vi "PRAMMS-LISTENER.vi"(0 "PRAMMS-COMM IN":refnum<visa-resource-name>="Yp\u0000\u0002", 1 "Bool Refnum":refnum<vi>, 2 "MessageTypeArray":cluster{string[], u32[]}={["emtError", "emtAreYouThere", "emtAcknowledgment", "emtGetClientType", "emtClientType", "emtGetImageExposureTime", "emtSetImageExposureTime", "emtImageExposureTime", "emtGetOptimalExposureTime", "emtSetOptimalExposureTime", "emtOptimalExposureTime", "emtGetImageEMGain", "emtSetImageEMGain", "emtImageEMGain", "emtGetFPGACtrl", "emtSetFPGACtrl", "emtFPGACtrl", "emtGetImageWidth", "emtSetImageWidth", "emtImageWidth", "emtGetImageHeight", "emtSetImageHeight", "emtImageHeight", "emtGetImageBinning", "emtSetImageBinning", "emtImageBinning", "emtGetImageDisplayFrameRate", "emtSetImageDisplayFrameRate", "emtImageDisplayFrameRate", "emtGetROIWidth", "emtSetROIWidth", "emtROIWidth", "emtGetROIHeight", "emtSetROIHeight", "emtROIHeight", "emtGetROIXOffset", "emtSetROIXOffset", "emtROIXOffset", "emtGetROIYOffset", "emtSetROIYOffset", "emtROIYOffset", "emtStartAcquisition", "mtStopAcquisition", "emtAcquisitionStarted", "emtAcquisitionStopped", "emtGetFalconImage", "emtFalconImage"], [1, 2, 3, 4, 5, 1001, 1101, 1201, 1002, 1102, 1202, 1003, 1103, 1203, 1004, 1104, 1204, 1005, 1105, 1205, 1006, 1106, 1206, 1007, 1107, 1207, 1008, 1108, 1208, 1009, 1109, 1209, 1010, 1110, 1210, 1011, 1111, 1211, 1012, 1112, 1212, 1130, 1131, 1150, 1151, 1070, 1270]}, 7 "Signature":u32=1886544237, 11 "Error IN":errorcluster, 12 "ReadTimeOut":i32=5) -> (4 "PRAMMS-COMM OUT":refnum<visa-resource-name>, 6 "Type":string, 8 "Received":timestamp, 10 "ByteArray":u8[](array[numeric]), 14 "Received?":bool, 15 "Error OUT":errorcluster)   [LabVIEW 2019]
panel:
  out "DataReadTime":u32
  out "HeaderTime":u32
  out "Wait4FlagTime":u32=16
  out "MessageLength":u32
  out "CommandEnum":string[](array[string])=["emtError", "emtAreYouThere", "emtAcknowledgment", "emtGetClientType", "emtClientType", "emtGetImageExposureTime", "emtSetImageExposureTime", "emtImageExposureTime", "emtGetOptimalExposureTime", "emtSetOptimalExposureTime", "emtOptimalExposureTime", "emtGetImageEMGain", "emtSetImageEMGain", "emtImageEMGain", "emtGetFPGACtrl", "emtSetFPGACtrl", "emtFPGACtrl", "emtGetImageWidth", "emtSetImageWidth", "emtImageWidth", "emtGetImageHeight", "emtSetImageHeight", "emtImageHeight", "emtGetImageBinning", "emtSetImageBinning", "emtImageBinning", "emtGetImageDisplayFrameRate", "emtSetImageDisplayFrameRate", "emtImageDisplayFrameRate", "emtGetROIWidth", "emtSetROIWidth", "emtROIWidth", "emtGetROIHeight", "emtSetROIHeight", "emtROIHeight", "emtGetROIXOffset", "emtSetROIXOffset", "emtROIXOffset", "emtGetROIYOffset", "emtSetROIYOffset", "emtROIYOffset", "emtStartAcquisition", "mtStopAcquisition", "emtAcquisitionStarted", "emtAcquisitionStopped", "emtGetFalconImage", "emtFalconImage"]
  out "TypeEnum":u32[](array[numeric])=[1, 2, 3, 4, 5, 1001, 1101, 1201, 1002, 1102, 1202, 1003, 1103, 1203, 1004, 1104, 1204, 1005, 1105, 1205, 1006, 1106, 1206, 1007, 1107, 1207, 1008, 1108, 1208, 1009, 1109, 1209, 1010, 1110, 1210, 1011, 1111, 1211, 1012, 1112, 1212, 1130, 1131, 1150, 1151, 1070, 1270]
  # "Ce programme sera mis dans une boucle de communication \"ininterrompable\"\n\nIl doit toujours écouter la connexion si elle existe et retourne le EnumMessageTYpe\net le data string s'il existe.  Ainsi, quand il recevra un ACK, il retournera le code du\n\"emtAcknoledgment\" vers le programme principal qui s'occuppera de lever le flag.\n\nSon éxécution devra être suivi d'une boucle d'interprétation qui appelera le bon vi\nd'interprétation en fonction du MessageType reçu."
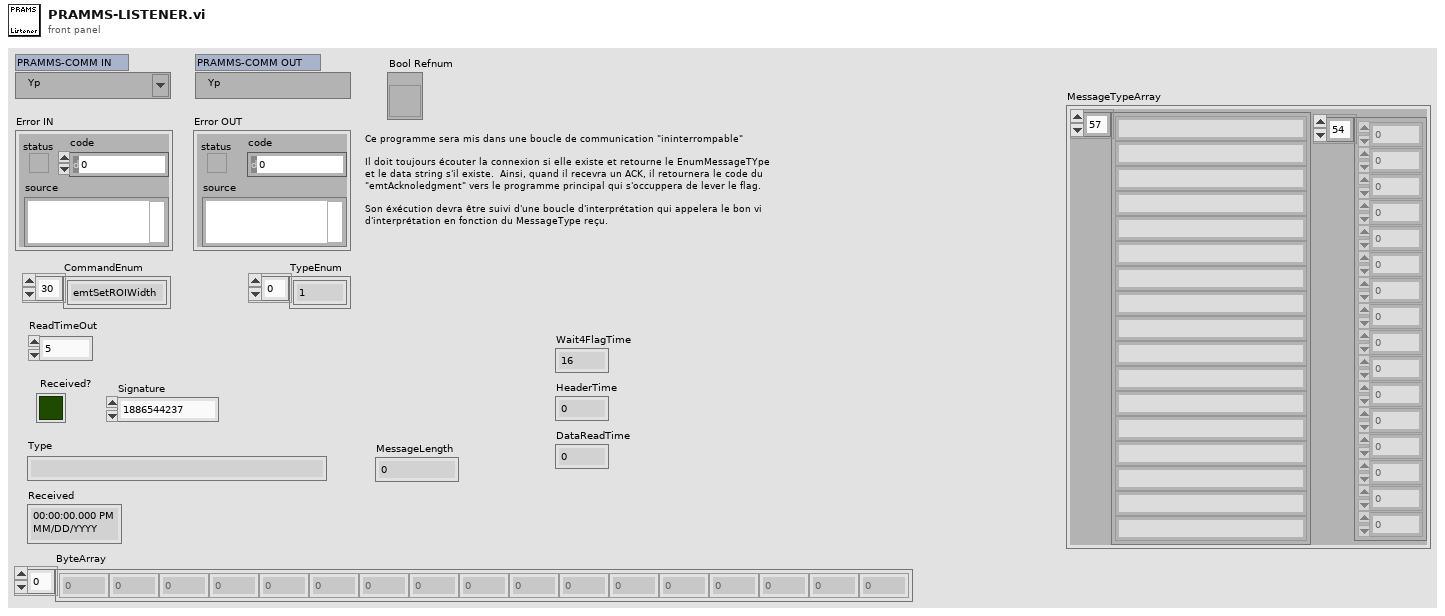
[diagram p1: front panel]
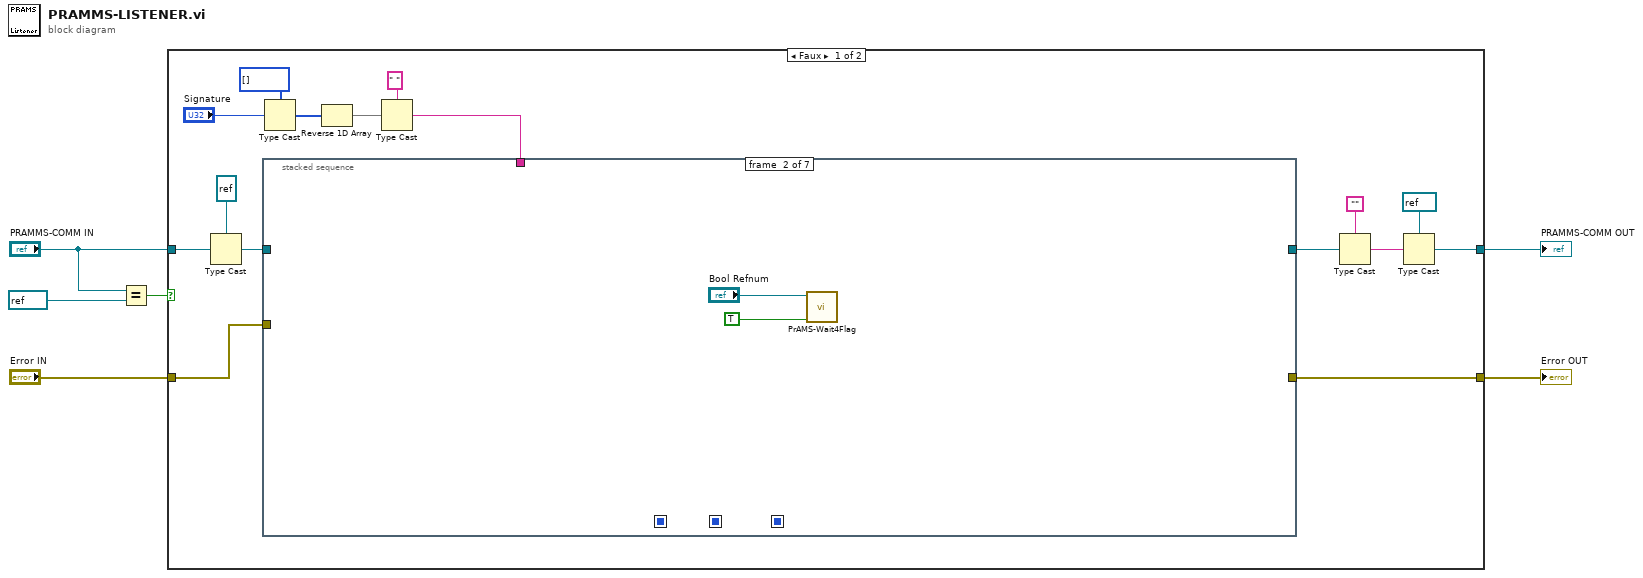
[diagram p0: block diagram]
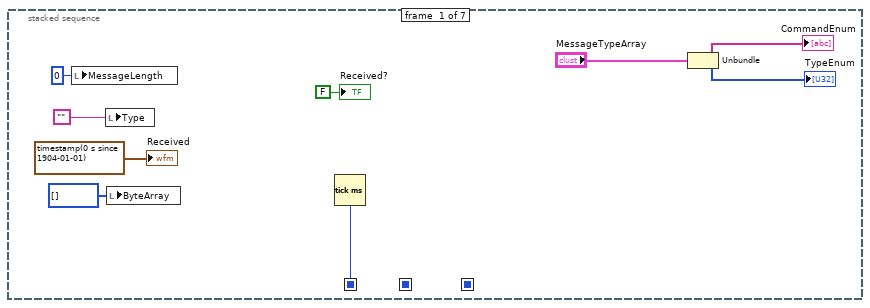
[diagram p2: hidden frame]
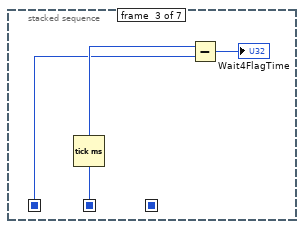
[diagram p3: hidden frame]
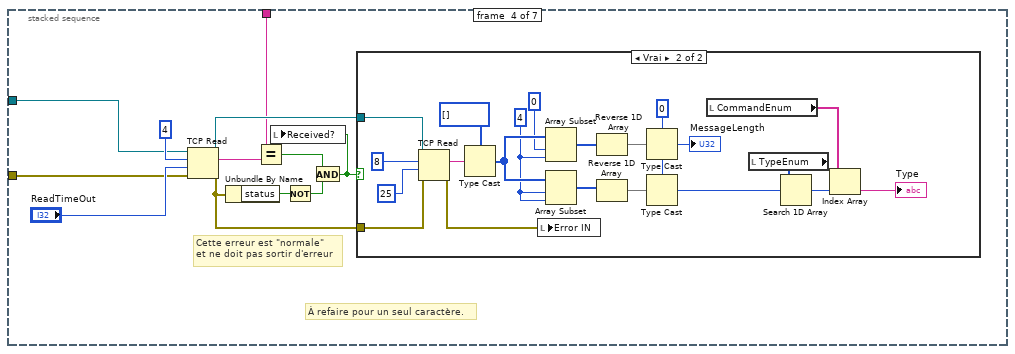
[diagram p4: hidden frame]
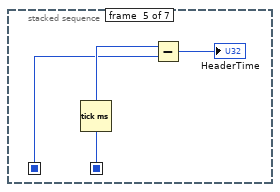
[diagram p6: hidden frame]
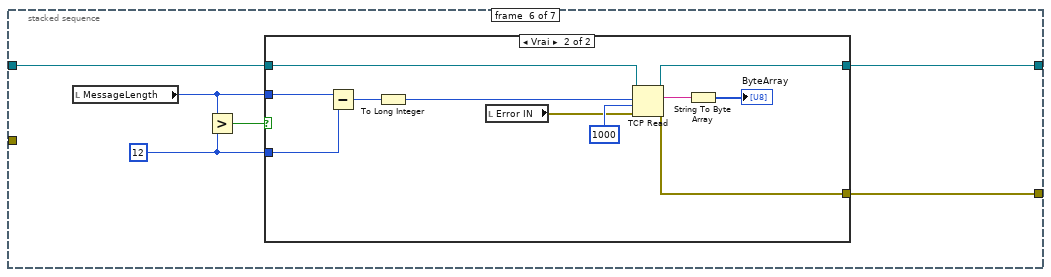
[diagram p7: hidden frame]
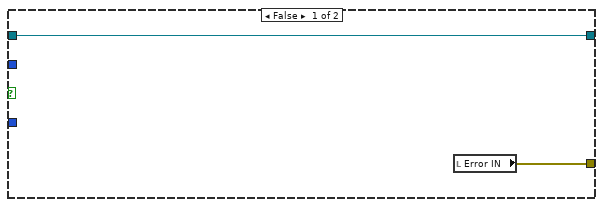
[diagram p8: hidden frame]
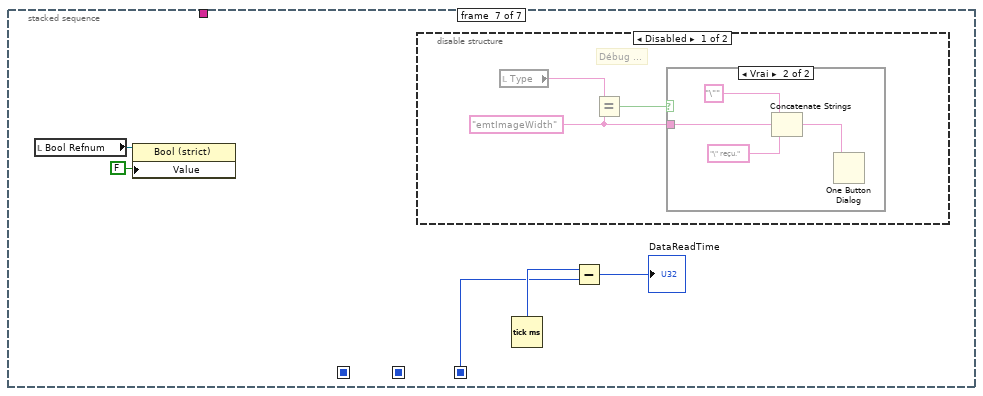
[diagram p9: hidden frame]
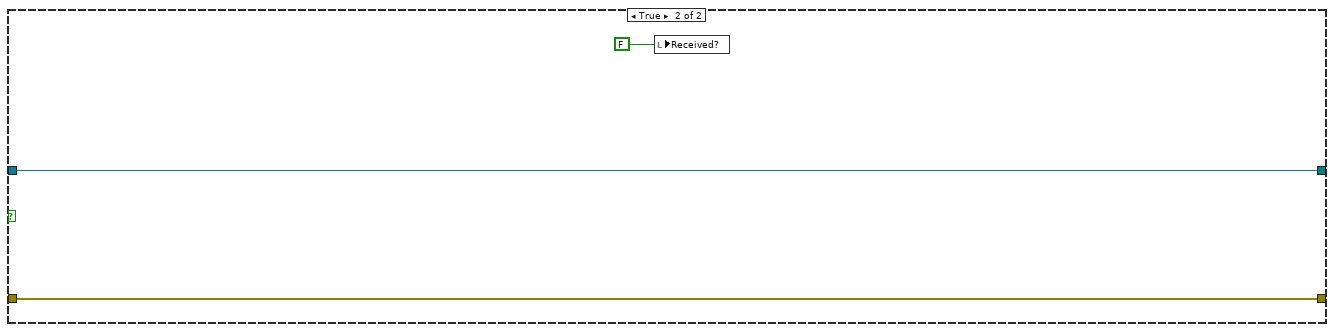
[diagram p12: hidden frame]
diagram:
  n1 = Equal?(x="PRAMMS-COMM IN", y=refnum<visa-resource-name> "-1") -> (x = y?=w5:bool)
  n2 = case shown="Faux" w5 {
    tunnel: "PRAMMS-COMM IN" -> [w22 w106]
    tunnel: "Error IN" -> [w19 w105]
    tunnel: [w14 w106] -> w1
    tunnel: [w18 w105] -> w2
    frame False {
      n3 = Type Cast(type=refnum<k5> refnum ("connection ID"), x=w22) -> (*(type *) &x=w21:refnum<k5>)
      n4 = Type Cast(type=u8[] [], x="Signature") -> (*(type *) &x=w12:u8[])
      n5 = Reverse 1D Array(array=w12) -> (reversed array=w9:u8[])
      n6 = Type Cast(type=" ", x=w9) -> (*(type *) &x=w7:string)
      n7 = stacked-sequence {
        seq-local: [w27 _ _ _ _ _ _] -> [_ _ w34 _ _ _ _]
        seq-local: [_ _ w35 _ _ _ _] -> [_ _ _ _ w70 _ _]
        seq-local: [_ _ _ _ w71 _ _] -> [_ _ _ _ _ _ w92]
        tunnel: w21 -> [_ _ _ w40 _ w75 _]
        tunnel: w19 -> [_ _ _ w39 _ _ _]
        tunnel: [_ _ _ _ _ w74 _] -> w18
        tunnel: [_ _ _ _ _ w73 _] -> w13
        tunnel: w7 -> [_ _ _ w38 _ _ _]
        frame #0 {
          n8 = local write "MessageLength"(u32 0 ("MessageLength")) -> ()
          n9 = local write "Type"("") -> ()
          n10 = local write "ByteArray"(u8[] [] ("ByteArray")) -> ()
          n11 = Tick Count (ms)() -> (millisecond timer value=w27:u32)
          n12 = Unbundle("MessageTypeArray") -> (→"CommandEnum":string[], →"TypeEnum":u32[])
          "Received?" <- FALSE ("RCV")
          "Received" <- timestamp(0 s since 1904-01-01) ("Received")
        }
        frame #1 {
          n13 = call "PrAMS-Wait4Flag.vi"("Raise Flag ?"=TRUE, "Ctl Refnum IN"="Bool Refnum") -> ()  [unwired: 8 in, 2 out]
        }
        frame #2 {
          n14 = Tick Count (ms)() -> (millisecond timer value=w35:u32)
          n15 = Subtract(x=w35, y=w34) -> (x-y=→"Wait4FlagTime":u32)
        }
        frame #3 {
          # "À refaire pour un seul caractère."
          # "Cette erreur est \"normale\"\net ne doit pas sortir d'erreur"
          n16 = TCP Read(connection ID=w40, bytes to read=4, error in (no error)=w39, 9:"ReadTimeOut") -> (connection ID out=w42:refnum<k5>, data out=w46:string, error out=w43:errorcluster)  [unwired: 1 in]
          n17 = Unbundle By Name(w43) -> ("status"=w44:bool)
          n18 = Equal?(x=w38, y=w46) -> (x = y?=w45:bool)
          n19 = Not(x=w44) -> (.not. x?=w37:bool)
          n20 = And(x=w45, y=w37) -> (x .and. y?=w41:bool)
          n21 = local write "Received?"(w41) -> ()
          n22 = case shown="Vrai" w41 {
            tunnel: w43 -> [_ w68]
            tunnel: w42 -> [_ w69]
            frame False {
            }
            frame True {
              w56 = u32 0
              w60 = 4 ("length")
              n23 = TCP Read(connection ID=w69, bytes to read=8, error in (no error)=w68, 9:25 ("timeout ms (25000)")) -> (data out=w63:string, error out=w49:errorcluster)  [unwired: 1 in, 1 out]
              n24 = Type Cast(type=u8[] [], x=w63) -> (*(type *) &x=w61:u8[])
              n25 = local write "Error IN"(w49) -> ()
              n26 = Array Subset(array=w61, index=0, length=w60) -> (w64:u8[])
              n27 = Array Subset(array=w61, index=w60, length=w60) -> (w65:u8[])
              n28 = Reverse 1D Array(array=w64) -> (reversed array=w59:u8[])
              n29 = Reverse 1D Array(array=w65) -> (reversed array=w57:u8[])
              n30 = Type Cast(type=w56, x=w59) -> (*(type *) &x=→"MessageLength":u32)
              n31 = Type Cast(type=w56, x=w57) -> (*(type *) &x=w54:u32)
              n32 = local read "CommandEnum"() -> (w52:string[])
              n33 = local read "TypeEnum"() -> (w53:u32[])
              n34 = Search 1D Array(1D array=w53, element=w54) -> (index of element=w50:i32)  [unwired: 1 in]
              n35 = Index Array(array=w52, index=w50) -> (element=→"Type":string)
            }
          }
        }
        frame #4 {
          n36 = Tick Count (ms)() -> (millisecond timer value=w71:u32)
          n37 = Subtract(x=w71, y=w70) -> (x-y=→"HeaderTime":u32)
        }
        frame #5 {
          w76 = u32 12 ("y")
          n38 = local read "MessageLength"() -> (w77:u32)
          n39 = Greater?(x=w77, y=w76) -> (0:w78:bool)
          n40 = case shown="Vrai" w78 {
            tunnel: w77 -> [_ w89]
            tunnel: w76 -> [_ w88]
            tunnel: w75 -> [w80 w83]
            tunnel: [w79 w82] -> w74
            tunnel: [w80 w81] -> w73
            frame False {
              n41 = local read "Error IN"() -> (w79:errorcluster)
            }
            frame True {
              n42 = Subtract(x=w89, y=w88) -> (x-y=w87:u32)
              n43 = To Long Integer(number=w87) -> (32bit integer=w86:i32)
              n44 = local read "Error IN"() -> (w90:errorcluster)
              n45 = TCP Read(connection ID=w83, bytes to read=w86, error in (no error)=w90, 9:1000 ("timeout ms (25000)")) -> (connection ID out=w81:refnum<k5>, data out=w85:string, error out=w82:errorcluster)  [unwired: 1 in]
              n46 = String To Byte Array(string=w85) -> (unsigned byte array=→"ByteArray":u8[])
            }
          }
        }
        frame #6 {
          n47 = local read "Bool Refnum"() -> (w95:refnum<vi>)
          n48 = property class="Bool (strict)"(reference=w95, "Value"=FALSE) -> ()  [unwired: 1 in, 2 out]
          n49 = disable-structure shown="Disabled" {
            frame Disabled {
              w97 = "emtImageWidth"
              # "Débug ..."
              n50 = local read "Type"() -> (w99:string)
              n51 = Equal?(x=w99, y=w97) -> (x = y?=w98:bool)
              n52 = case shown="Vrai" w98 {
                tunnel: w97 -> [_ w101]
                frame False {
                }
                frame True {
                  n53 = Concatenate Strings("\"" ("message"), w101, "\" reçu." ("message")) -> (w100:string)
                  n54 = One Button Dialog(message=w100) -> ()  [unwired: 1 in, 1 out]
                }
              }
            }
            frame Enabled {
            }
          }
          n55 = Tick Count (ms)() -> (millisecond timer value=w93:u32)
          n56 = Subtract(x=w93, y=w92) -> (x-y=→"DataReadTime":u32)
        }
      }
      n57 = Type Cast(type="", x=w13) -> (*(type *) &x=w15:string)
      n58 = Type Cast(type=refnum<visa-resource-name> refnum ("y"), x=w15) -> (*(type *) &x=w14:refnum<visa-resource-name>)
    }
    frame True {
      n59 = local write "Received?"(FALSE ("RCV")) -> ()
    }
  }
  "Error OUT" <- w2
  "PRAMMS-COMM OUT" <- w1
